vi "Main.vi"() -> ()   [LabVIEW 2016]
uses:
  <vilib>/Analysis/Matrix/Datatypes/RealMatrix.ctl
  AndyLabview/stateType.ctl
  <vilib>/Utility/error.llb/DialogType.ctl
  <vilib>/DAQmx/read.llb/DAQmx Read (Analog 2D DBL NChan NSamp).vi
  <vilib>/Analysis/baseanly.llb/A x Vector.vi
  <vilib>/Instr/_visa.llb/VISA Configure Serial Port (Instr).vi
  <vilib>/DAQmx/miscellaneous.llb/DAQmx Fill In Error Info.vi
  <vilib>/Analysis/Matrix/Numeric/Conversions/Array To Matrix - RA.vi
  <vilib>/Utility/file.llb/Write Delimited Spreadsheet (DBL).vi
  <userlib>/dynamixel32bit/dynamixel.lvlib
  <vilib>/Analysis/NI_AALBase.lvlib
  <vilib>/Analysis/Matrix/NI_Matrix.lvlib
panel:
  in  "Servo Execution\nTime (ms)":dbl
  in  "Sweep Angle Cmd (rad/s)":dbl
  in  "Rotation Speed (rad/s)":dbl
  in  "Gantry Y Velocity (cm/s)":dbl
  in  "Gantry X Velocity (cm/s)":dbl
  out "Total F/T Waveform":dbl[][](graph)
  in  "Save Out Force Data?":bool=TRUE
  in  "Data Out Filename":path
  out "Force Units":string
  out "Torque Units":string
  in  "Tool Transform":T1
  in  "Calibration File":path=path "D:/YasBed/Mini40Calib/FT24266/FT24266.cal"
  in  "First A# Channel":i16=1
  in  "Device Num : DAQ Card":tag="Dev1"
  in  "Maximum Value":dbl=10.0 caption="Maximum Value (V)" format="%0.2f"
  in  "Minimum Value":dbl=-10.0 caption="Minimum Value (V)" format="%0.2f"
  in  "Sample Rate":dbl=10000.0 caption="Sample Rate (Hz)" format="%0.2f"
  in  "Serial Input:\nSetX;SetY;SetZ":string
  in  "Gantry Board (Due) VISA":refnum<visa-resource-name>="COM15"
  in  "Tilt Board (Uno) VISA":refnum<visa-resource-name>="COM17"
  out "Global time (ms)":u32
  out "Current State":T2
  in  "Desired Bed \nAngle (deg)":string="0"
  out "Voltages":dbl[][](array[numeric])
  in  "Bias FTT":bool
  out "Bias Vector (V)":dbl[](array[numeric])
  in  "Unbias FTT":bool
  in  "Samples to Read":i32=1000
  out "Instant F/T Waveform":dbl[][](graph)
  in  "stop 2":bool caption="stop"
  out "F/T":T3
  out "Tilt Angle (deg)":dbl
  in  "stop":bool
  out "Present Position":u16(slide) max=1023 scale=0.0..1023.0
  out "Rotator Motor Position V. Time":i32(graph)
  in  "Rotator Dynamixel ID":i32=1
  in  "Wheel Dynamixel ID":i32=1
  in  "Wheel Speed":u16=512 max=1023 step=1
  in  "Theta Naught":dbl
  in  "Angle Increment per Step":dbl
  in  "# of Steps per Gait Cycle":dbl
  in  "Baud Rate":i32=1
  in  "Com Port":i32=3
  in  "Step Delay (Seconds)":dbl
  out "Wheel Motor Position V. Time 3":i32(graph)
  # "Motor Control"
  # "Initialization"
  # "COM 16"
  # "ID 12"
  # "Baud 1"
  # "ID 6"
  # "Motor Parameters"
  # "Example: 256 + 12(21.333) = 512"
  # "256"
  # "+"
  # "21.333"
  # "x"
  # "12"
  # "= 512"
  # "Common Values by Gait:\n     Wave Gait:\n          Step Delay:\n          Theta Naught:\n          Angle Increment:\n          # of Steps/cycle:\n     RP Gait:\n          Step Delay:\n          Theta Naught:\n          Angle Increment:\n          # of Steps/cycle:\n     Rear Rotator Pedaling Gait:\n          Step Delay:\n          Theta Naught:\n          Angle Increment:\n          # of Steps/cycle:"
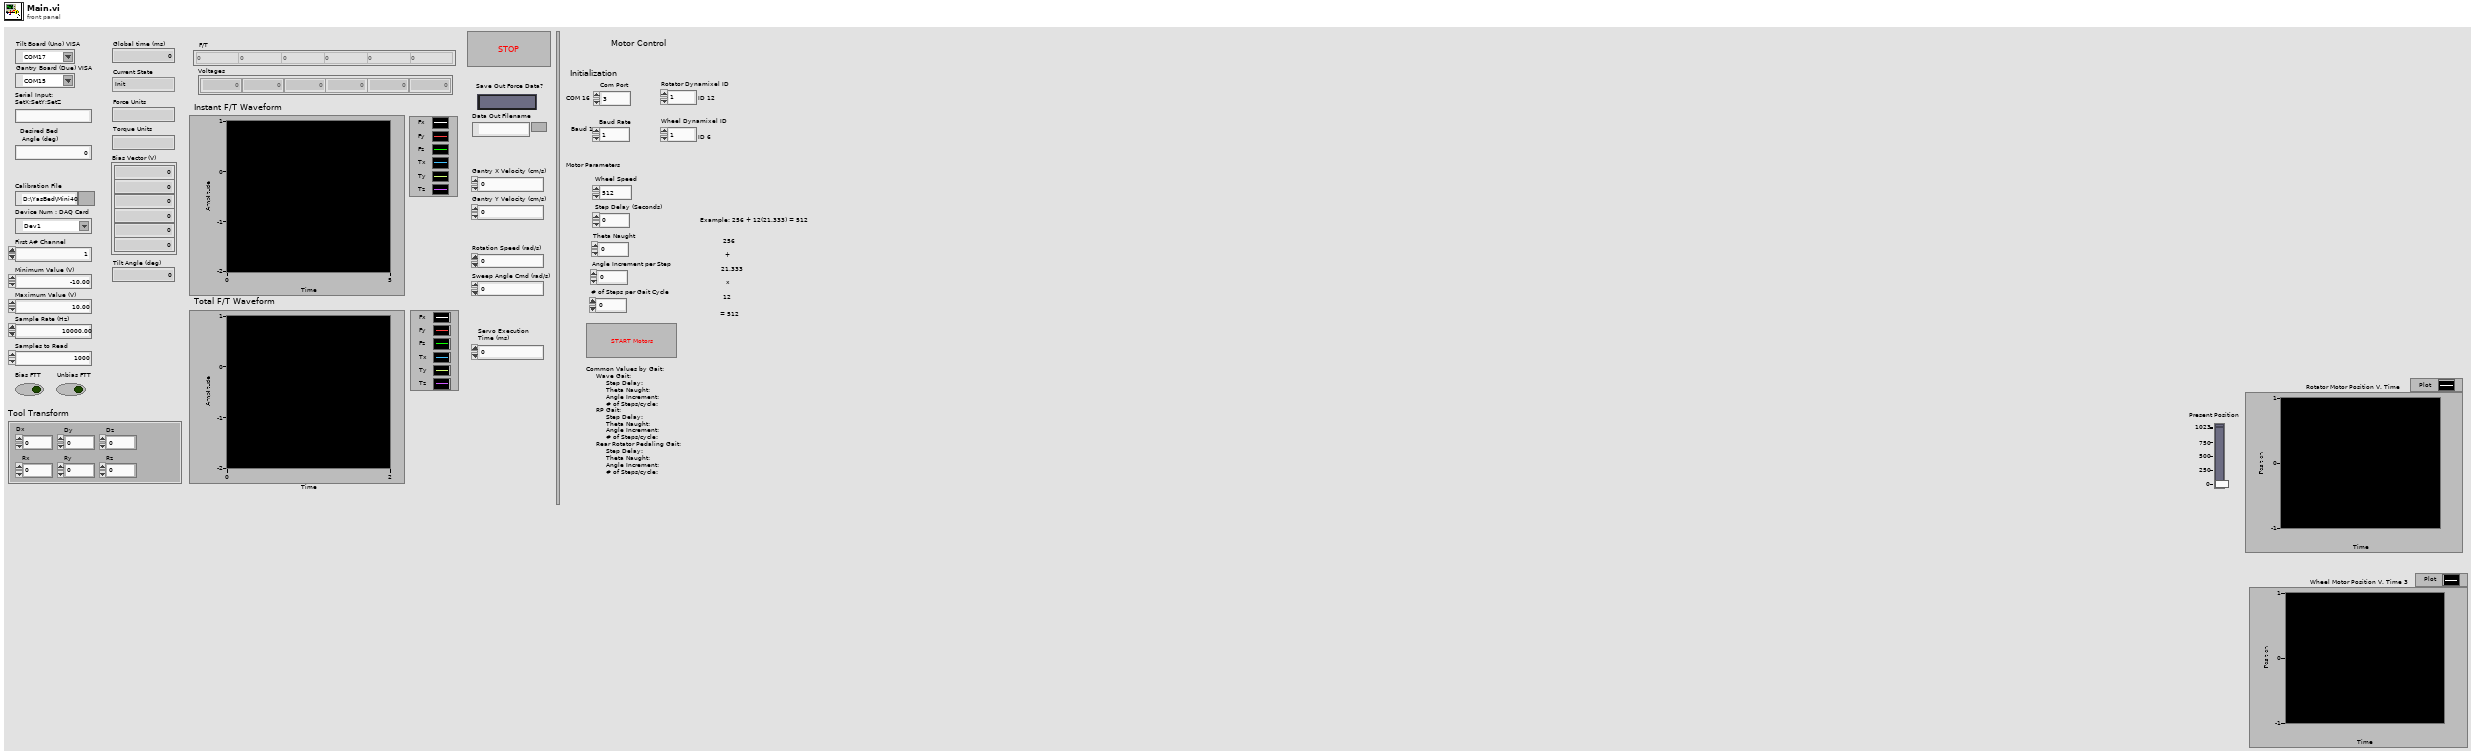
[diagram p1: front panel]
types:
  T1 = cluster{"Dx":dbl, "Dy":dbl, "Dz":dbl, "Rx":dbl, "Ry":dbl, "Rz":dbl}
  T2 = typedef "stateType.ctl" = enum16{"Init", "Standby", "Set XY", "Engage Tilt", "Set Z", "Do Main", "Retract Z", "Reset Tilt", "Fluidize", "Save", "Exit"}
  T3 = typedef "NI_Matrix.lvlib/RealMatrix.ctl" = dbl[][]
  T4 = typedef "DialogType.ctl" = u16
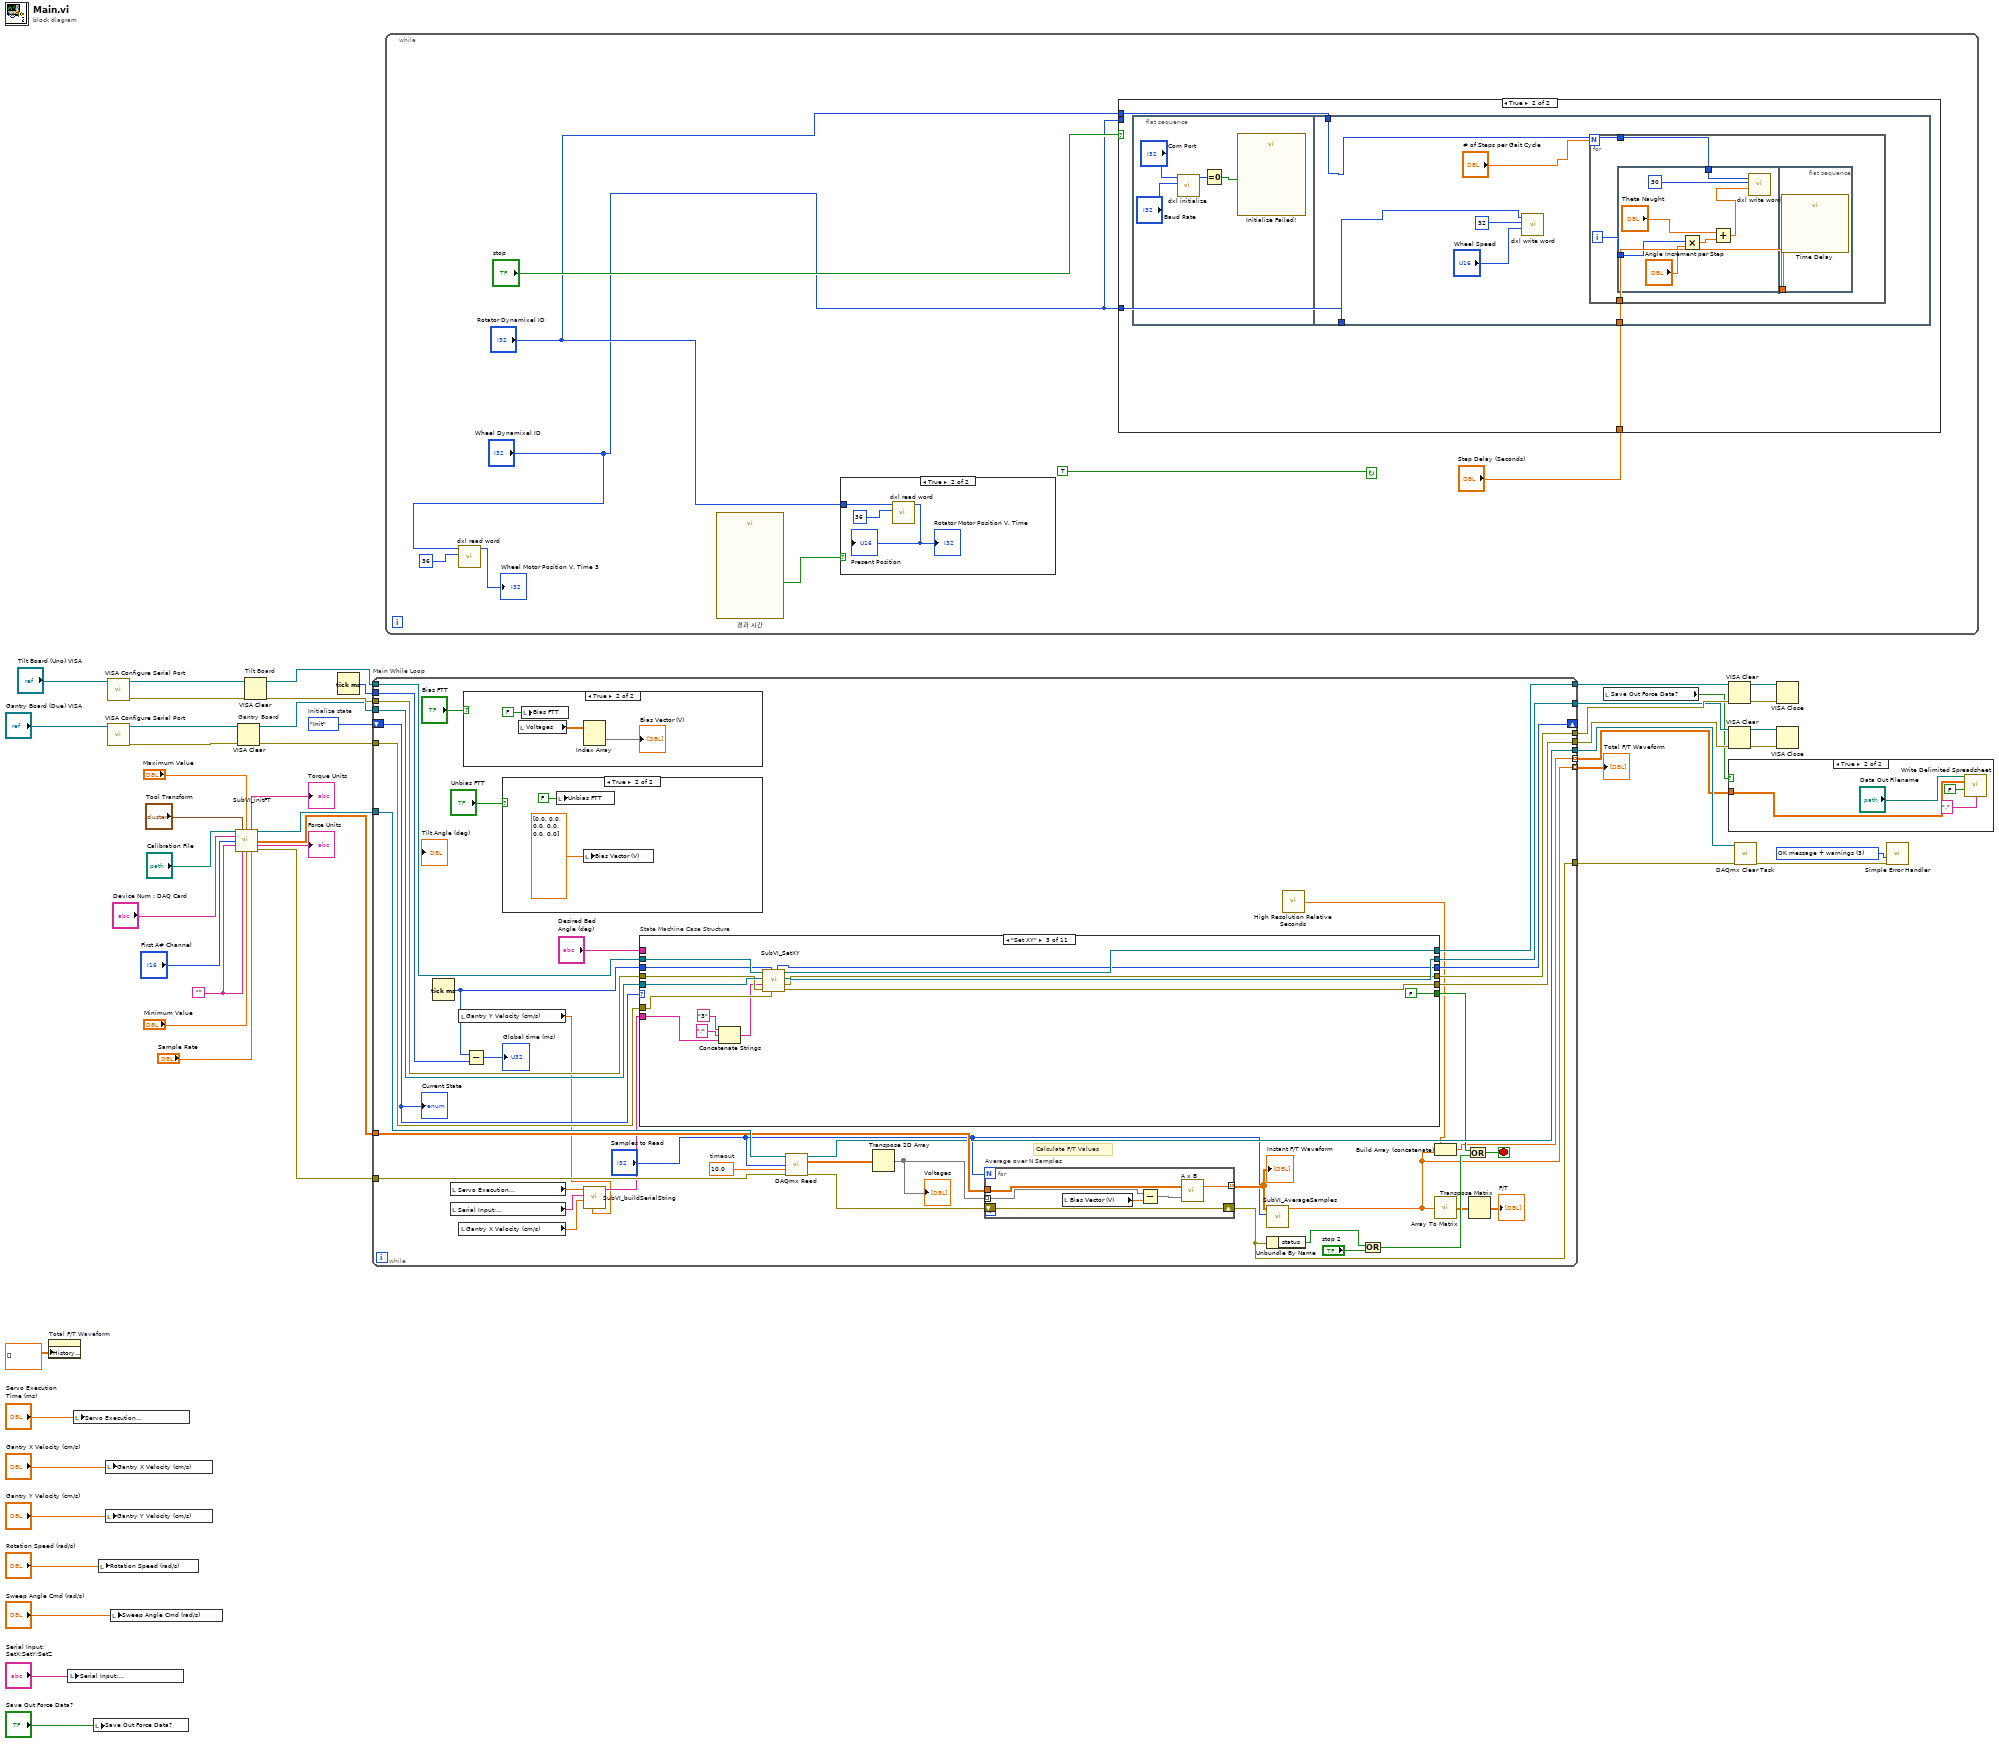
[diagram p0: block diagram]
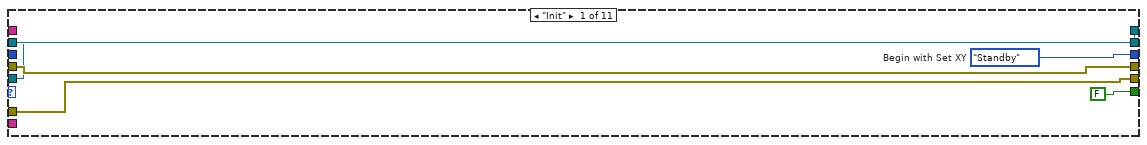
[diagram p5: hidden frame]
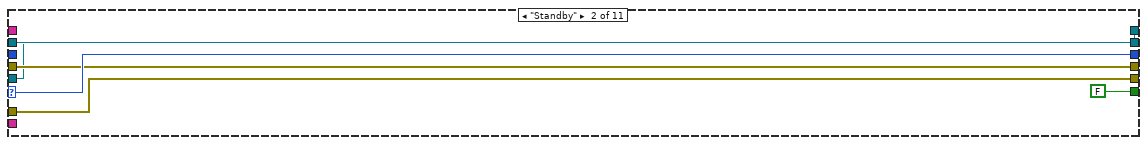
[diagram p6: hidden frame]
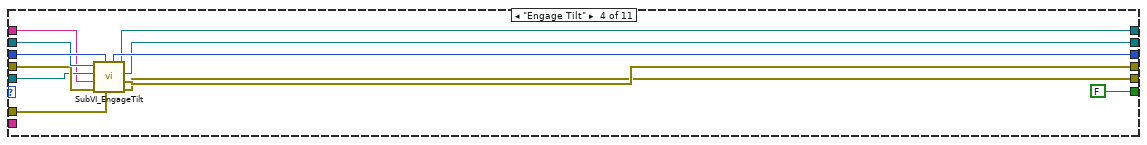
[diagram p7: hidden frame]
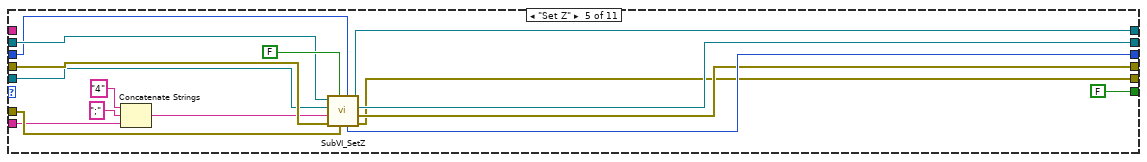
[diagram p8: hidden frame]
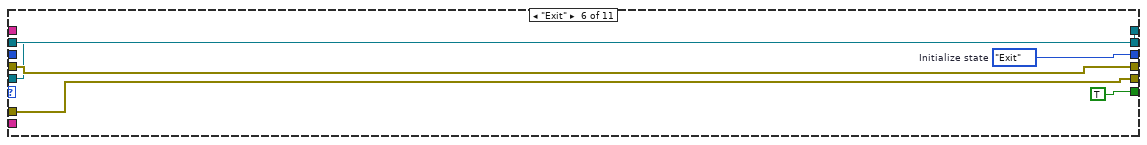
[diagram p9: hidden frame]
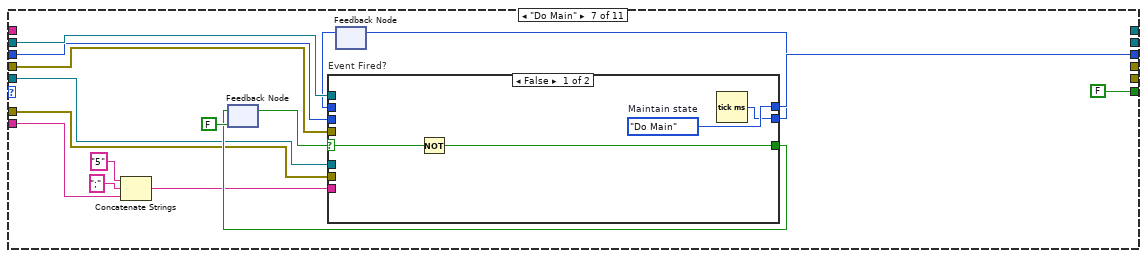
[diagram p10: hidden frame]
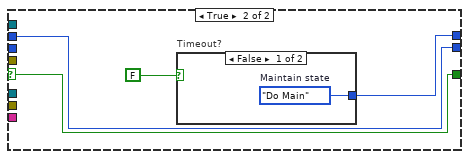
[diagram p11: hidden frame]
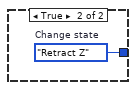
[diagram p12: hidden frame]
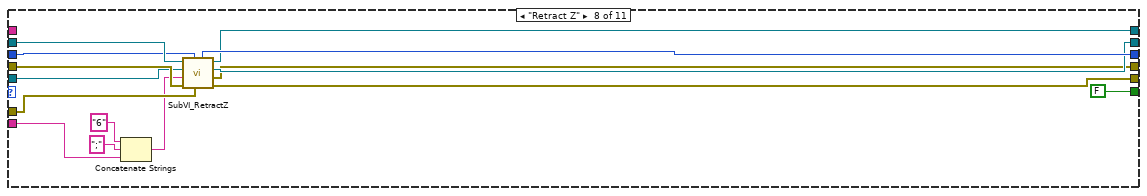
[diagram p13: hidden frame]
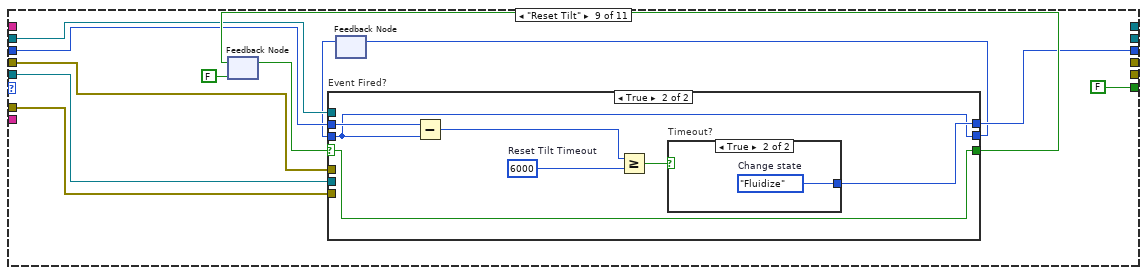
[diagram p14: hidden frame]
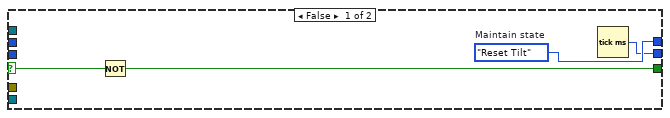
[diagram p15: hidden frame]
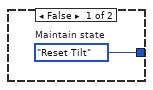
[diagram p16: hidden frame]
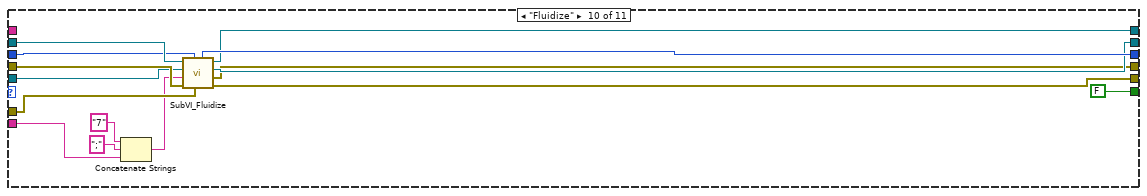
[diagram p17: hidden frame]
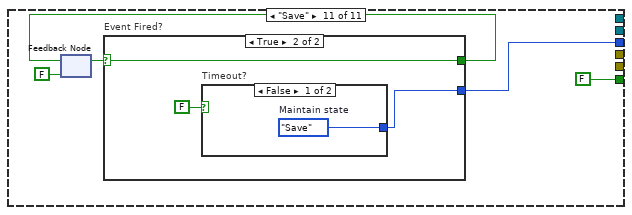
[diagram p18: hidden frame]
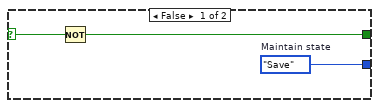
[diagram p19: hidden frame]
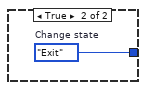
[diagram p20: hidden frame]
diagram:
  w21 = T4 3 items=["no dialog", "OK message", "continue or stop message", "OK message + warnings", "continue/stop + warnings"] ("type of dialog (OK msg:1)")
  w23 = ""
  w48 = stateType."Init"  # Initialize state
  n1 = property on="Total F/T Waveform" class="WFChart (strict)"("History Data"=dbl[][] []) -> ()  [unwired: 2 in, 2 out]
  n2 = local write "Serial Input:\nSetX;SetY;SetZ"("Serial Input:\nSetX;SetY;SetZ") -> ()
  n3 = local write "Servo Execution\nTime (ms)"("Servo Execution\nTime (ms)") -> ()
  n4 = local write "Save Out Force Data?"("Save Out Force Data?") -> ()
  n5 = local write "Rotation Speed (rad/s)"("Rotation Speed (rad/s)") -> ()
  n6 = local write "Gantry X Velocity (cm/s)"("Gantry X Velocity (cm/s)") -> ()
  n7 = local write "Gantry Y Velocity (cm/s)"("Gantry Y Velocity (cm/s)") -> ()
  n8 = call-poly "VISA Configure Serial Port"("VISA resource name"="Tilt Board (Uno) VISA") -> ("VISA resource name out"=w45:refnum<visa-resource-name>, "error out"=w44:errorcluster)  [unwired: 13 in]
  n9 = call-poly "VISA Configure Serial Port"("VISA resource name"="Gantry Board (Due) VISA") -> ("VISA resource name out"=w41:refnum<visa-resource-name>, "error out"=w40:errorcluster)  [unwired: 13 in]
  n10 = local write "Sweep Angle Cmd (rad/s)"("Sweep Angle Cmd (rad/s)") -> ()
  n11 = call "SubVI_initFT.vi"("Calibration File"="Calibration File", "Transform"="Tool Transform", "Maximum Value"="Maximum Value", "DAQ Card"="Device Num : DAQ Card", "First Channel"="First A# Channel", "Torque Units in"=w23, "Force Units in"=w23, "Minimum Value"="Minimum Value", "Sample Rate"="Sample Rate") -> ("Torque Units out"=→"Torque Units":string, "Refnum out"=w25:refnum<k21>, "Transformed Calibration Matrix"=w26:dbl[][], "Force Units out"=→"Force Units":string, "error out"=w24:errorcluster)  [unwired: 1 in, 1 out]
  n12 = VISA Clear "Gantry Board"(VISA resource name=w41, error in (no error)=w40) -> (VISA resource name out=w39:refnum<visa-resource-name>, error out=w38:errorcluster)
  n13 = VISA Clear "Tilt Board"(VISA resource name=w45, error in (no error)=w44) -> (VISA resource name out=w43:refnum<visa-resource-name>, error out=w42:errorcluster)
  n14 = Tick Count (ms)() -> (millisecond timer value=w37:u32)
  n15 = while "Main While Loop" {
    shift-right: [w89] -> _
    shift-left: w48 -> [w90]
    tunnel: w39 -> [w84]
    tunnel: w38 -> [w82]
    tunnel: w43 -> [w88]
    tunnel: w42 -> [w86]
    tunnel: [w87] -> w14
    tunnel: [w85] -> w13
    tunnel: [w83] -> w12
    tunnel: [w81] -> w11
    tunnel: w37 -> [w80]
    tunnel: w26 -> [w70]
    tunnel: w25 -> [w72]
    tunnel: w24 -> [w71]
    tunnel: [w68] -> w20
    tunnel: [w65] -> w19
    tunnel: [w58] -> w4 mode=indexing
    tunnel: [w54] -> w3 mode=indexing
    stop <- w62 stop-if-true
    w75 = 10.0  # timeout
    # "Calculate F/T Values"
    n16 = Tick Count (ms)() -> (millisecond timer value=w79:u32)
    n17 = local read "Servo Execution\nTime (ms)"() -> (w49:dbl)
    n18 = local read "Serial Input:\nSetX;SetY;SetZ"() -> (w53:string)
    n19 = local read "Gantry Y Velocity (cm/s)"() -> (w50:dbl)
    n20 = local read "Gantry X Velocity (cm/s)"() -> (w51:dbl)
    n21 = case shown="True" "Bias FTT" {
      frame False {
      }
      frame True {
        n22 = local read "Voltages"() -> (w101:dbl[][])
        n23 = local write "Bias FTT"(FALSE) -> ()
        n24 = Index Array(array=w101) -> (element=→"Bias Vector (V)":dbl[])  [unwired: 2 in]
      }
    }
    n25 = Subtract(x=w79, y=w80) -> (x-y=→"Global time (ms)":u32)
    n26 = case shown="True" "Unbias FTT" {
      frame False {
      }
      frame True {
        n27 = local write "Unbias FTT"(FALSE) -> ()
        n28 = local write "Bias Vector (V)"(dbl[] [0.0, 0.0, 0.0, 0.0, 0.0, 0.0]) -> ()
      }
    }
    n29 = call "SubVI_buildSerialString.vi"("Gantry Y Velocity (cm/s)"=w50, "Gantry X Velocity (cm/s)"=w51, "Serial Input:\nSetX;SetY;SetZ"=w53, "Servo Execution\nTime (ms)"=w49) -> ("String"=w52:string)  [unwired: 7 in]
    n30 = case "State Machine Case Structure" shown="\"Set XY\"" w90 {
      selector: w90 -> [_ w113 _ _ _ _ _ _ _ _ _]
      tunnel: [w107 w113 w119 w140 w155 w162 w175 w203 w212 w243 w245] -> w89
      tunnel: [FALSE FALSE FALSE FALSE FALSE TRUE FALSE FALSE FALSE FALSE FALSE] -> w63
      tunnel: [w106 w112 w122 w137 w145 w160 _ w191 _ w231 _] -> w87
      tunnel: w88 -> [w106 w112 w124 w138 w153 w160 w173 w201 w210 w241 _]
      tunnel: [w105 w111 w121 w135 w144 w159 _ w190 _ w230 _] -> w85
      tunnel: w86 -> [w105 w111 w123 w136 w152 w159 w172 w200 w209 w240 _]
      tunnel: w84 -> [w104 w110 w128 w134 w151 w158 w171 w199 w208 w239 _]
      tunnel: [w104 w110 w126 w132 w143 w158 _ w193 _ w233 _] -> w83
      tunnel: w82 -> [w103 w109 w127 w133 w150 w157 w170 w198 w207 w238 _]
      tunnel: [w103 w109 w125 w131 w142 w157 _ w192 _ w232 _] -> w81
      tunnel: w79 -> [_ _ w120 w139 w141 _ w163 w189 w206 w229 _]
      tunnel: w52 -> [_ _ w115 _ w147 _ w167 w195 _ w235 _]
      tunnel: "Desired Bed \nAngle (deg)" -> [_ _ _ w129 _ _ _ _ _ _ _]
      frame "Init" {
        w107 = stateType."Standby"  # Begin with Set XY
      }
      frame "Standby" {
      }
      frame "Set XY" {
        n31 = Concatenate Strings("3", ";", w115) -> (w114:string)
        n32 = call "SubVI_SetXY.vi"("error out 4"=w127, "millisecond timer value"=w120, "error in (no error)"=w123, "String"=w114, "VISA resource name out 4"=w128, "VISA Refnum in"=w124) -> (0:"error out"=w125:errorcluster, 1:"error out"=w121:errorcluster, "VISA resource name out 3"=w126:refnum<visa-resource-name>, "VISA Refnum out"=w122:refnum<visa-resource-name>, "Change state"=w119:T2)  [unwired: 1 in]
      }
      frame "Engage Tilt" {
        n33 = call "SubVI_EngageTilt.vi"("error in"=w133, "millisecond timer value"=w139, "error in (no error)"=w136, "Desired Bed \nAngle (deg)"=w129, "VISA resource name in"=w134, "VISA Refnum in"=w138) -> ("error out"=w131:errorcluster, "error out 3"=w135:errorcluster, "VISA resource name out"=w132:refnum<visa-resource-name>, "VISA Refnum out"=w137:refnum<visa-resource-name>, "Change state"=w140:T2)  [unwired: 1 in]
      }
      frame "Set Z" {
        n34 = Concatenate Strings("4", ";", w147) -> (w146:string)
        n35 = call "SubVI_SetZ.vi"("millisecond timer value"=w141, "error out 3"=w150, "Boolean"=FALSE, "error in (no error)"=w152, "String"=w146, "VISA resource name out 3"=w151, "VISA Refnum in"=w153) -> ("error out"=w142:errorcluster, "error out 2"=w144:errorcluster, "VISA resource name out"=w143:refnum<visa-resource-name>, "VISA Refnum out"=w145:refnum<visa-resource-name>, "Change state"=w155:T2)
      }
      frame "Exit" {
        w162 = stateType."Exit"  # Initialize state
      }
      frame "Do Main" {
        n36 = Concatenate Strings("5", ";", w167) -> (w166:string)
        n37 = feedback #1(FALSE) -> (w177:bool)
        n38 = feedback #2() -> (w164:u32)  [unwired: 1 in]
        n39 = case "Event Fired?" shown="False" w177 {
          selector: w177 -> [w182 w186]
          tunnel: [w181 w186] -> w176
          tunnel: [w180 w185] -> w175
          tunnel: w173 -> [_ _]
          tunnel: w172 -> [_ _]
          tunnel: w171 -> [_ _]
          tunnel: w170 -> [_ _]
          tunnel: w166 -> [_ _]
          tunnel: w164 -> [_ w184]
          tunnel: [w179 w184] -> w165
          tunnel: w163 -> [_ _]
          frame False {
            w180 = stateType."Do Main"  # Maintain state
            n40 = Not(x=w182) -> (.not. x?=w181:bool)
            n41 = Tick Count (ms)() -> (millisecond timer value=w179:u32)
          }
          frame True {
            n42 = case "Timeout?" shown="False" FALSE {
              tunnel: [w187 w188] -> w185
              frame False {
                w187 = stateType."Do Main"  # Maintain state
              }
              frame True {
                w188 = stateType."Retract Z"  # Change state
              }
            }
          }
        }
        n43 = feedback-in #1(w176) -> ()
        n44 = feedback-in #2(w165) -> ()
      }
      frame "Retract Z" {
        n45 = Concatenate Strings("6", ";", w195) -> (w194:string)
        n46 = call "SubVI_RetractZ.vi"("error out 3"=w198, "millisecond timer value"=w189, "error in (no error)"=w200, "String"=w194, "VISA resource name out 3"=w199, "VISA Refnum in"=w201) -> (0:"error out"=w192:errorcluster, 1:"error out"=w190:errorcluster, "VISA resource name out 2"=w193:refnum<visa-resource-name>, "VISA Refnum out"=w191:refnum<visa-resource-name>, "Change state"=w203:T2)  [unwired: 1 in]
      }
      frame "Reset Tilt" {
        n47 = feedback #3(FALSE) -> (w214:bool)
        n48 = feedback #4() -> (w204:u32)  [unwired: 1 in]
        n49 = case "Event Fired?" shown="True" w214 {
          selector: w214 -> [w219 w226]
          tunnel: [w218 w226] -> w213
          tunnel: [w217 w225] -> w212
          tunnel: w210 -> [_ _]
          tunnel: w209 -> [_ _]
          tunnel: w208 -> [_ _]
          tunnel: w207 -> [_ _]
          tunnel: w206 -> [_ w224]
          tunnel: w204 -> [_ w223]
          tunnel: [w216 w223] -> w205
          frame False {
            w217 = stateType."Reset Tilt"  # Maintain state
            n50 = Not(x=w219) -> (.not. x?=w218:bool)
            n51 = Tick Count (ms)() -> (millisecond timer value=w216:u32)
          }
          frame True {
            w221 = u32 6000  # Reset Tilt Timeout
            n52 = Subtract(x=w224, y=w223) -> (x-y=w222:u32)
            n53 = Greater Or Equal?(x=w222, y=w221) -> (x >= y?=w220:bool)
            n54 = case "Timeout?" shown="True" w220 {
              tunnel: [w227 w228] -> w225
              frame False {
                w227 = stateType."Reset Tilt"  # Maintain state
              }
              frame True {
                w228 = stateType."Fluidize"  # Change state
              }
            }
          }
        }
        n55 = feedback-in #3(w213) -> ()
        n56 = feedback-in #4(w205) -> ()
      }
      frame "Fluidize" {
        n57 = Concatenate Strings("7", ";", w235) -> (w234:string)
        n58 = call "SubVI_Fluidize.vi"("error out 3"=w238, "millisecond timer value"=w229, "error in (no error)"=w240, "String"=w234, "VISA resource name out 3"=w239, "VISA Refnum in"=w241) -> (0:"error out"=w232:errorcluster, 1:"error out"=w230:errorcluster, "VISA resource name out 2"=w233:refnum<visa-resource-name>, "VISA Refnum out"=w231:refnum<visa-resource-name>, "Change state"=w243:T2)  [unwired: 1 in]
      }
      frame "Save" {
        n59 = feedback #5(FALSE) -> (w247:bool)
        n60 = case "Event Fired?" shown="True" w247 {
          selector: w247 -> [w251 w254]
          tunnel: [w250 w254] -> w246
          tunnel: [w249 w253] -> w245
          frame False {
            w249 = stateType."Save"  # Maintain state
            n61 = Not(x=w251) -> (.not. x?=w250:bool)
          }
          frame True {
            n62 = case "Timeout?" shown="False" FALSE {
              tunnel: [w255 w256] -> w253
              frame False {
                w255 = stateType."Save"  # Maintain state
              }
              frame True {
                w256 = stateType."Exit"  # Change state
              }
            }
          }
        }
        n63 = feedback-in #5(w246) -> ()
      }
    }
    n64 = call-poly <vilib>:"DAQmx Read.vi"("task/channels in"=w72, "number of samples per channel"="Samples to Read", "timeout"=w75, "error in"=w71) -> ("task out"=w68:refnum<k21>, "data"=w73:dbl[][], "error out"=w74:errorcluster)  [unwired: 9 in]
    n65 = Transpose 2D Array(2D array=w73) -> (transposed array=w69:dbl[][])
    "Voltages" <- w69
    n66 = for "Average over N Samples" {
      N: "Samples to Read" -> [_]
      tunnel: [w93] -> w61 mode=indexing
      shift-right: [w92] -> w65
      shift-left: w74 -> [w92]
      tunnel: w69 -> [w96] mode=indexing
      tunnel: w70 -> [w91]
      n67 = local read "Bias Vector (V)"() -> (w95:dbl[])
      n68 = Subtract(x=w96, y=w95) -> (x-y=w94:dbl[])
      n69 = call-poly <vilib>:"A x B.vi"("Vector"=w94, "A"=w91) -> ("A x Vector"=w93:dbl[])  [unwired: 1 out]
    }
    "Instant F/T Waveform" <- w61
    n70 = call "SubVI_AverageSamples.vi"("Samples to Read"="Samples to Read", "Input Samples Matrix"=w61) -> ("Single Valued Signal Out"=w54:dbl[])  [unwired: 9 in]
    n71 = Unbundle By Name(w65) -> ("status"=w66:bool)
    n72 = call <vilib>:"High Resolution Relative Seconds.vi"() -> ("relative seconds"=w56:dbl)
    n73 = Or(x=w66, y="stop 2") -> (x .or. y?=w64:bool)
    n74 = Build Array (concatenate)(w56, w54) -> (w58:dbl[])
    n75 = call-poly <vilib>:"Array To Matrix.vi"("Real 1D Array"=w54) -> ("Real Matrix (Column Vector)"=w59:T3)
    n76 = Or(x=w63, y=w64) -> (x .or. y?=w62:bool)
    n77 = Transpose Matrix(1:w59) -> (0:→"F/T":T3)
    "Current State" <- w90
  }
  "Total F/T Waveform" <- w3
  n78 = while {
    stop <- TRUE continue-if-true
    n79 = call <userlib>:"dxl read word.vi"("address"=36, "id"="Wheel Dynamixel ID") -> ("function return"=→"Wheel Motor Position V. Time 3":i32)  [unwired: 9 in]
    n80 = call "경과 시간"() -> ("Time has Elapsed"=w263:bool)  [unwired: 12 in, 7 out]
    n81 = case shown="True" w263 {
      tunnel: "Rotator Dynamixel ID" -> [_ w294]
      frame False {
      }
      frame True {
        n82 = call <userlib>:"dxl read word.vi"("address"=36, "id"=w294) -> ("function return"=→"Present Position" →"Rotator Motor Position V. Time":i32)  [unwired: 9 in]
      }
    }
    n83 = case shown="True" "stop" {
      tunnel: "Wheel Dynamixel ID" -> [w266 _]
      tunnel: "Rotator Dynamixel ID" -> [_ w270]
      tunnel: "Wheel Dynamixel ID" -> [_ w269]
      tunnel: "Step Delay (Seconds)" -> [_ w268]
      frame False {
        n84 = call <userlib>:"dxl write word.vi"("value"=0, "address"=32, "id"=w266) -> ()  [unwired: 9 in]
      }
      frame True {
        n85 = flat-sequence {
          tunnel: w270 -> [w278]
          tunnel: w269 -> [w277]
          tunnel: w268 -> [w276]
          frame #0 {
            n86 = call <userlib>:"dxl initialize.vi"("baudnum"="Baud Rate", "devIndex"="Com Port") -> ("function return"=w273:i32)  [unwired: 9 in]
            n87 = Equal To 0?(x=w273) -> (x = 0?=w274:bool)
            n88 = call "Initialize Failed!"("Enable"=w274) -> ()  [unwired: 9 in, 2 out]
          }
          frame #1 {
            n89 = call <userlib>:"dxl write word.vi"("value"="Wheel Speed", "address"=32, "id"=w277) -> ()  [unwired: 9 in]
            n90 = for {
              N: "# of Steps per Gait Cycle" -> [_]
              tunnel: w278 -> [w283]
              tunnel: w276 -> [w281]
              i -> [w282]
              n91 = flat-sequence {
                tunnel: w283 -> [w289]
                tunnel: w282 -> [w288]
                tunnel: w281 -> [w291]
                frame #0 {
                  n92 = Multiply(x=w288, y="Angle Increment per Step") -> (x*y=w287:dbl)
                  n93 = Add(x="Theta Naught", y=w287) -> (x+y=w286:dbl)
                  n94 = call <userlib>:"dxl write word.vi"("value"=w286, "address"=30, "id"=w289) -> ()  [unwired: 9 in]
                }
                frame #1 {
                  n95 = call "Time Delay"("Delay Time (s)"=w291) -> ()  [unwired: 10 in, 1 out]
                }
              }
            }
          }
        }
      }
    }
  }
  n96 = local read "Save Out Force Data?"() -> (w9:bool)
  n97 = VISA Clear(VISA resource name=w14, error in (no error)=w13) -> (VISA resource name out=w16:refnum<visa-resource-name>, error out=w15:errorcluster)
  n98 = VISA Clear(VISA resource name=w12, error in (no error)=w11) -> (VISA resource name out=w18:refnum<visa-resource-name>, error out=w17:errorcluster)
  n99 = case shown="True" w9 {
    tunnel: w4 -> [_ w297]
    frame False {
    }
    frame True {
      n100 = call-poly <vilib>:"Write Delimited Spreadsheet.vi"("file path (dialog if empty)"="Data Out Filename", "2D data"=w297, "append to file? (new file:F)"=FALSE, "delimiter (\\t)"=",") -> ()  [unwired: 10 in, 2 out]
    }
  }
  n101 = call <vilib>:"DAQmx Clear Task.vi"("task in"=w20, "error in"=w19) -> ("error out"=w22:errorcluster)  [unwired: 13 in]
  n102 = VISA Close(VISA resource name=w16, error in (no error)=w15) -> ()  [unwired: 1 out]
  n103 = VISA Close(VISA resource name=w18, error in (no error)=w17) -> ()  [unwired: 1 out]
  n104 = call <vilib>:"Simple Error Handler.vi"("type of dialog (OK msg:1)"=w21, "error in (no error)"=w22) -> ()  [unwired: 3 in, 5 out]
